vi "set colour mode.vi"(8 "error in (no error)":errorcluster, 11 "Thorcam in":refnum<class "Thorcam.lvclass">) -> (0 "error out":errorcluster, 3 "Thorcam out":refnum<class "Thorcam.lvclass">)   [LabVIEW 2012, in "Thorcam.lvclass"]
uses:
  Thorcam.lvclass
  Thorcam.lvclass/Thorcam.ctl
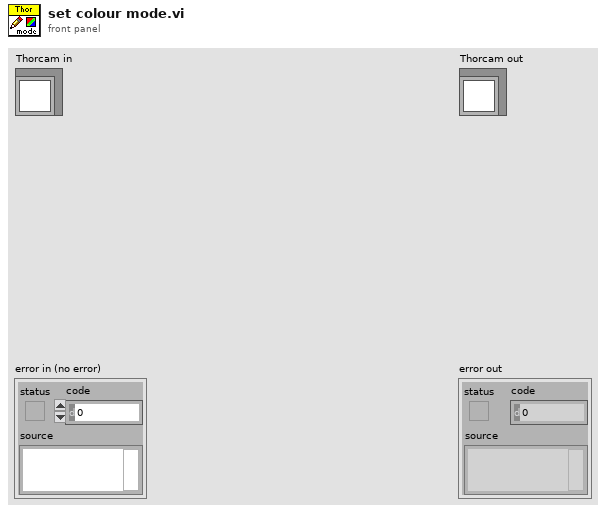
[diagram p1: front panel]
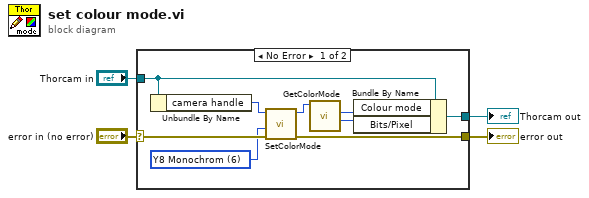
[diagram p0: block diagram]
diagram:
  n1 = case shown="No Error" "error in (no error)" {
    selector: "error in (no error)" -> [w12 w15]
    tunnel: [w11 w15] -> w3
    tunnel: [w7 w14] -> w1
    tunnel: "Thorcam in" -> [w8 w14]
    frame No Error {
      w10 = 6 items=["RGB 32"=0, "RGB 24"=1, "Y8 Monochrom"=6] ("Mode")
      n2 = Unbundle By Name(w8) -> ("camera handle"=w13:u32)
      n3 = call <instrlib>:"SetColorMode.vi"("error in"=w12, "Mode"=w10, "Camera Handle In"=w13) -> ("error out"=w11:errorcluster, "Camera Handle Out"=w9:u32)  [unwired: 7 in]
      n4 = call <instrlib>:"GetColorMode.vi"("Camera Handle In"=w9) -> ("Bits/Pixel"=w6:i32, "ColorMode"=w5:i32)  [unwired: 8 in, 1 out]
      n5 = Bundle By Name(cluster=w8, "Colour mode"=w5, "Bits/Pixel"=w6) -> (w7:refnum<class "Thorcam.lvclass">)
    }
    frame Error {
    }
  }
  "error out" <- w3
  "Thorcam out" <- w1
